vi "Global_UI.vi"() -> ()   [LabVIEW 2013]
panel:
  in  "Variable References":cluster{"Output Values":refnum<k21>}
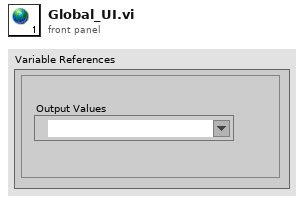
[diagram p1: front panel]
diagram:
